vi "get parameter - array of bytes.vi"(6 "buffer size (256)":i32=256, 8 "error in (no error)":errorcluster, 10 "parameter":u8 format="%x", 11 "channel":u16 format="%x") -> (0 "error out":errorcluster)   [LabVIEW 2024, in "atsj peakcan basic.lvlib"]
doc: "Gets a parameter from a PeakCAN <b>channel</b>."
uses:
  atsj peakcan basic.lvlib
  support/x64/PCANBasic.dll
panel:
  out "value":u8[](array[numeric])
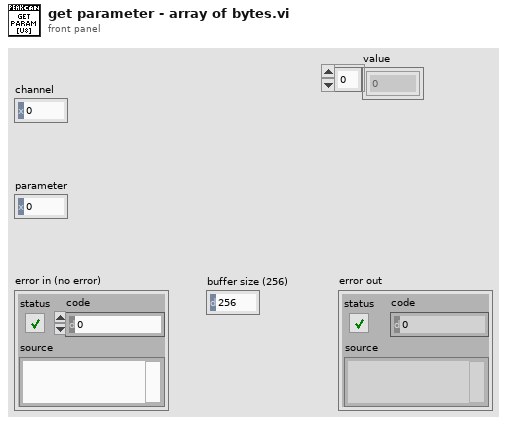
[diagram p1: front panel]
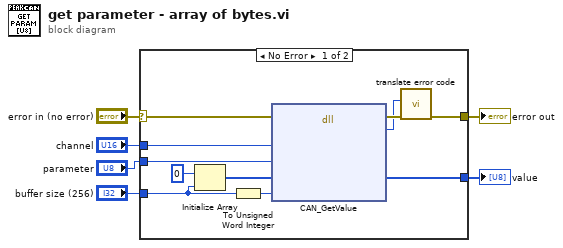
[diagram p0: block diagram]
diagram:
  n1 = case shown="No Error" "error in (no error)" {
    selector: "error in (no error)" -> [w11 w18]
    tunnel: [w12 w18] -> w5
    tunnel: [w13 _] -> w1
    tunnel: "channel" -> [w10 _]
    tunnel: "parameter" -> [w9 _]
    tunnel: "buffer size (256)" -> [w8 _]
    frame No Error {
      n2 = Initialize Array(u8 0, w8) -> (w7:u8[])
      n3 = To Unsigned Word Integer(number=w8) -> (unsigned 16bit integer=w15:u16)
      n4 = dll-call lib="C:/atsj/plateau/atsj-peakcan-basic-for-labview/src/support/x64/PCANBasic.dll" fn="CAN_GetValue" ("get parameter - array of bytes")(error in=w11, "Channel"=w10, "Parameter"=w9, "Buffer"=w7, "BufferLength"=w15) -> (error out=w17:errorcluster, "Status"=w16:u32, "Buffer"=w13:u8[])  [unwired: 5 in, 1 out]
      n5 = call "translate error code.vi"("error in (no error)"=w17, "error code"=w16) -> ("error out"=w12:errorcluster)  [unwired: 9 in]
    }
    frame Error {
    }
  }
  "error out" <- w5
  "value" <- w1
